vi "Configure Trigger Source.vi"(8 "error in (no error)":errorcluster, 10 "Trigger Source(0)":u16(ring) items=["MANUal", "BUS"], 11 "VISA resource name":refnum<visa-resource-name>) -> (0 "error out":errorcluster, 3 "VISA resource name out":refnum<visa-resource-name>)   [LabVIEW 2020, in "IT6500.lvlib"]
doc: "This command selects the source of the trigger signal.The power supply can receive the trigger signal from the panel (keyboard trigger <b>Trigger</b> key) or receive a bus Trigger signal."
uses:
  IT6500.lvlib
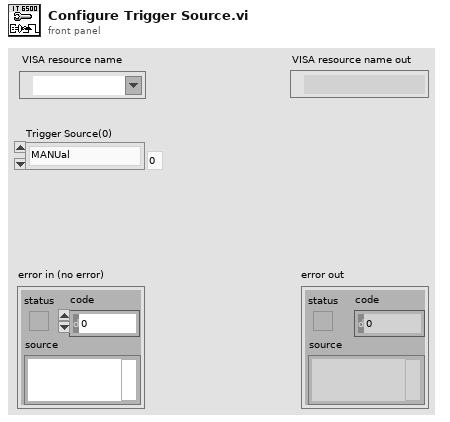
[diagram p1: front panel]
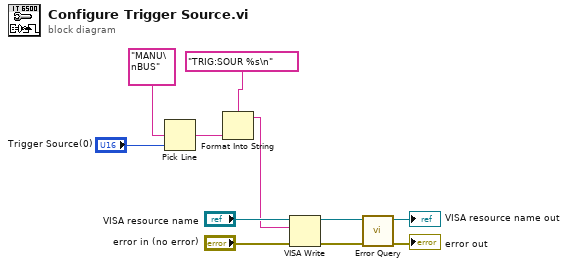
[diagram p0: block diagram]
diagram:
  n1 = Pick Line(multi-line string="MANU\nBUS", line index="Trigger Source(0)") -> (output string=w1:string)  [unwired: 1 in]
  n2 = Format Into String(format string="TRIG:SOUR %s\n", w1) -> (resulting string=w3:string)  [unwired: 2 in, 1 out]
  n3 = VISA Write(VISA resource name="VISA resource name", write buffer=w3, error in (no error)="error in (no error)") -> (VISA resource name out=w8:refnum<visa-resource-name>, error out=w9:errorcluster)  [unwired: 1 out]
  n4 = call "Error Query.vi"("error in (no error)"=w9, "VISA resource name"=w8) -> ("error out"=→"error out":errorcluster, "VISA resource name out"=→"VISA resource name out":refnum<visa-resource-name>)  [unwired: 6 in, 2 out]
